vi "SR830ReadOutRef.vi"(3 "error in (no error)":errorcluster, 4 "ReadOut (1: Voltage Amplitude)":u16(ring)=1 items=["Voltage Out (Vrms)"=1, "Frequency (Hz)"=2, "Aux Out 1 (VDC)"=3, "Aux Out 2 (VDC)"=4, "Time Constant (s)"=5, "Roll-Off Slope (dB/oct)"=6], 5 "VISA resource name":refnum<visa-resource-name>) -> (0 "error out":errorcluster, 1 "ReadOut":dbl, 2 "VISA resource name out":refnum<visa-resource-name>)   [LabVIEW 2016]
uses:
  <instrlib>/Stanford Research 830/Stanford Research 830.lvlib
panel:
  # "This VI reads reference values from the SR830 Lock-in Amplifier using GPIB\nIncluded parameters to choose from are Sine out Voltage, Frequency, Aux out1, Aux out 2, and time constant"
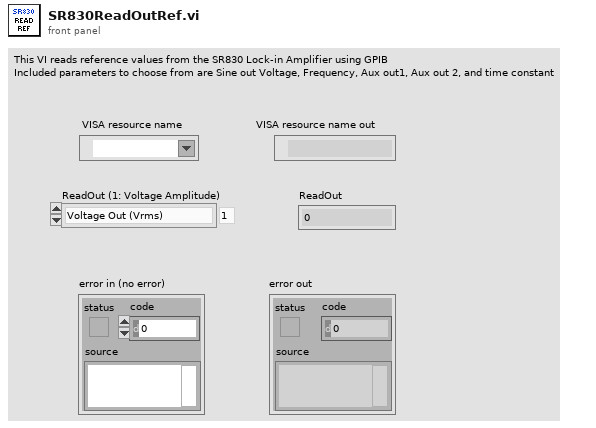
[diagram p1: front panel]
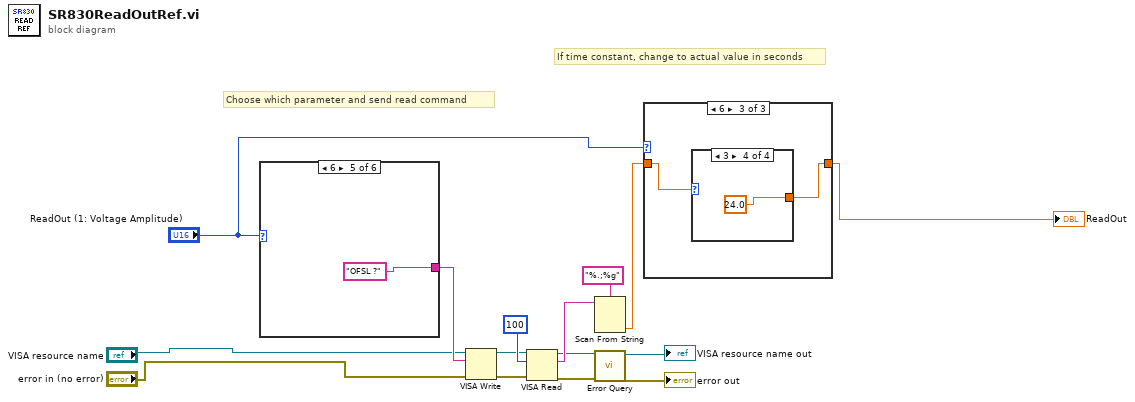
[diagram p0: block diagram]
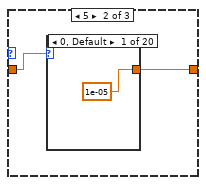
[diagram p3: hidden frame]
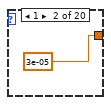
[diagram p4: hidden frame]
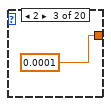
[diagram p5: hidden frame]
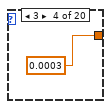
[diagram p6: hidden frame]
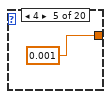
[diagram p7: hidden frame]
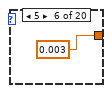
[diagram p8: hidden frame]
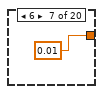
[diagram p9: hidden frame]
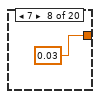
[diagram p10: hidden frame]
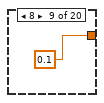
[diagram p11: hidden frame]
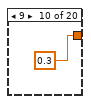
[diagram p12: hidden frame]
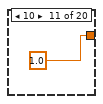
[diagram p13: hidden frame]
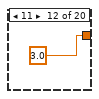
[diagram p14: hidden frame]
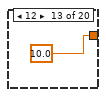
[diagram p15: hidden frame]
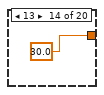
[diagram p16: hidden frame]
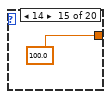
[diagram p17: hidden frame]
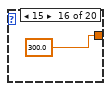
[diagram p18: hidden frame]
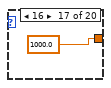
[diagram p19: hidden frame]
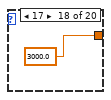
[diagram p20: hidden frame]
diagram:
  # "If time constant, change to actual value in seconds"
  # "Choose which parameter and send read command"
  n1 = case shown="6" "ReadOut (1: Voltage Amplitude)" {
    tunnel: ["FREQ ? " ("string (\"\")") "AUXV ? 1" ("string (\"\")") "AUXV ? 2" ("string (\"\")") "OFLT ?" ("string (\"\")") "OFSL ?" ("string (\"\")") "SLVL ? " ("string (\"\")")] -> w13
    frame 2 {
    }
    frame 3 {
    }
    frame 4 {
    }
    frame 5 {
    }
    frame 6 {
    }
    frame 1, Default {
    }
  }
  n2 = VISA Write(VISA resource name="VISA resource name", write buffer=w13, error in (no error)="error in (no error)") -> (VISA resource name out=w7:refnum<visa-resource-name>, error out=w6:errorcluster)  [unwired: 1 out]
  n3 = VISA Read(VISA resource name=w7, byte count=u32 100, error in (no error)=w6) -> (VISA resource name out=w9:refnum<visa-resource-name>, read buffer=w15:string, error out=w8:errorcluster)  [unwired: 1 out]
  n4 = Scan From String(format string="%.;%g", input string=w15) -> (output 1=w3:dbl)  [unwired: 3 in, 3 out]
  n5 = call <instrlib>:"Error Query.vi"("error in (no error)"=w8, "VISA resource name"=w9) -> ("error out"=→"error out":errorcluster, "VISA resource name out"=→"VISA resource name out":refnum<visa-resource-name>)  [unwired: 7 in, 1 out]
  n6 = case shown="6" "ReadOut (1: Voltage Amplitude)" {
    tunnel: w3 -> [w22 w24 w46]
    tunnel: [w22 w23 w45] -> w2
    frame Default {
    }
    frame 5 {
      n7 = case shown="0, Default" w24 {
        tunnel: [1e-05 3e-05 0.0001 0.0003 0.001 0.003 0.01 0.03 0.1 0.3 1.0 3.0 10.0 30.0 100.0 300.0 1000.0 3000.0 10000.0 30000.0] -> w23
        frame 0, Default {
        }
        frame 1 {
        }
        frame 2 {
        }
        frame 3 {
        }
        frame 4 {
        }
        frame 5 {
        }
        frame 6 {
        }
        frame 7 {
        }
        frame 8 {
        }
        frame 9 {
        }
        frame 10 {
        }
        frame 11 {
        }
        frame 12 {
        }
        frame 13 {
        }
        frame 14 {
        }
        frame 15 {
        }
        frame 16 {
        }
        frame 17 {
        }
        frame 18 {
        }
        frame 19 {
        }
      }
    }
    frame 6 {
      n8 = case shown="3" w46 {
        tunnel: [6.0 12.0 18.0 24.0] -> w45
        frame 0, Default {
        }
        frame 1 {
        }
        frame 2 {
        }
        frame 3 {
        }
      }
    }
  }
  "ReadOut" <- w2
